vi "WriteHeader.vi"(0 "Path In":path, 1 "error in (no error)":errorcluster, 2 "Line 1":string, 3 "Line 2":string, 4 "Line 3":string, 5 "Line 4":string, 7 "Line 5":string, 8 "UTC format":bool, 9 "Line 6":string, 11 "Line 7":string, 13 "Line 8":string, 18 "Line 10":string, 19 "Line 9":string) -> (14 "Path":path, 17 "error out":errorcluster)   [LabVIEW 2009]
doc: "This VI takes a file path (required) and appends a 10 line header. Each line of the header can be specified separately.\nLines are first run through the Format Date String VI, so entries such as %H:%M will be interpreted correctly. This VI is an important part of \"StartLogfile.vi\""
uses:
  <vilib>/Utility/file.llb/Write To Spreadsheet File (string).vi
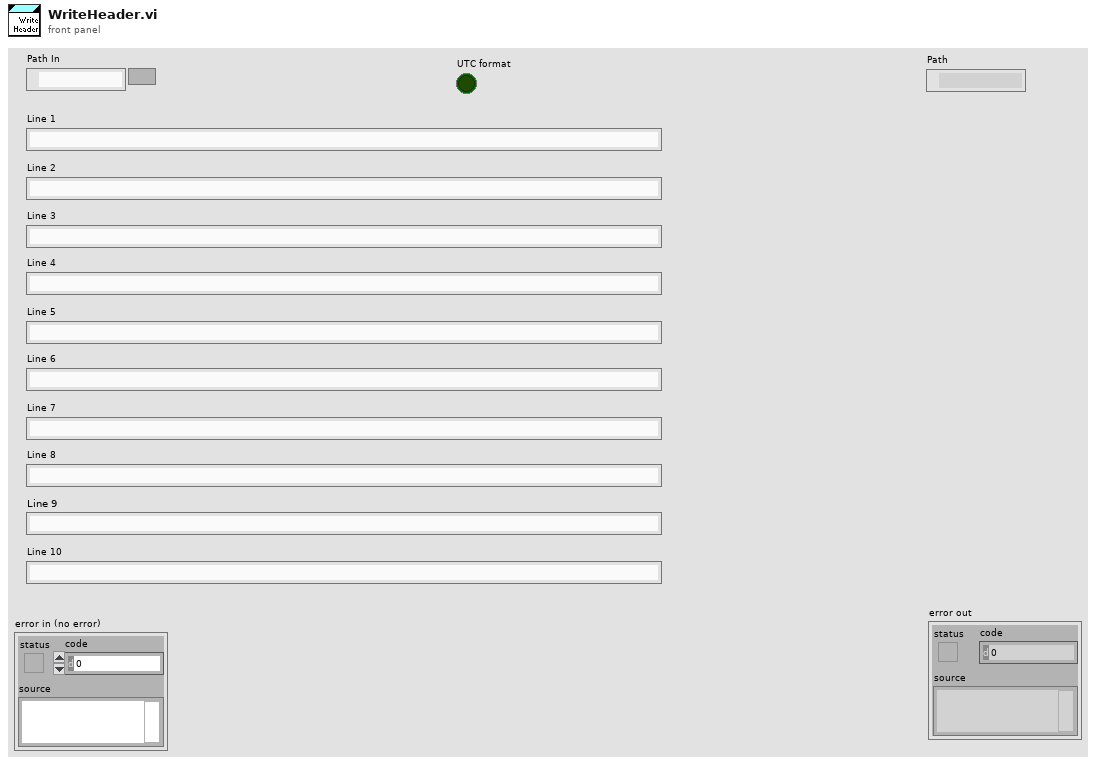
[diagram p1: front panel]
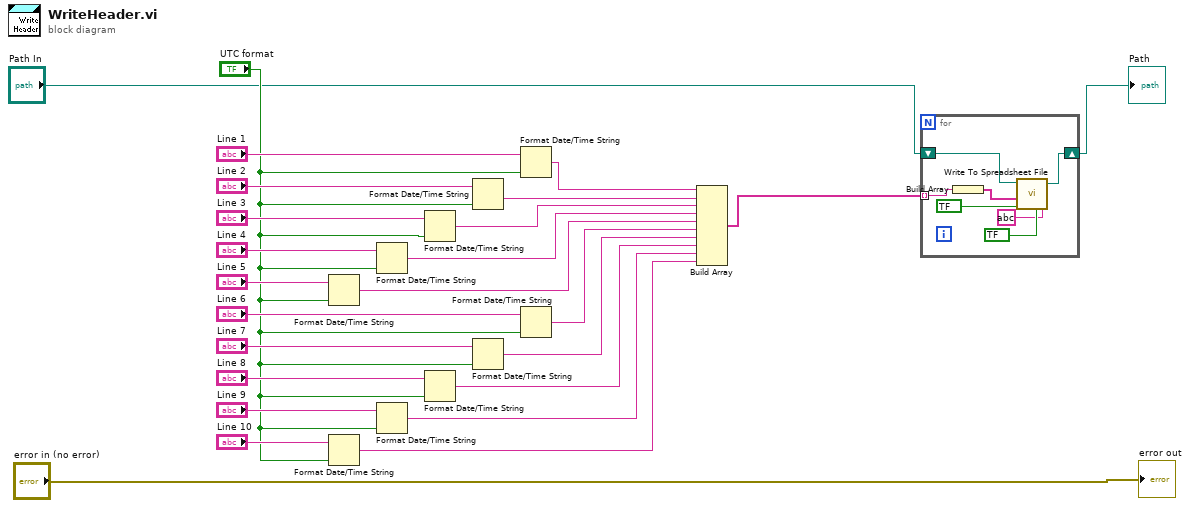
[diagram p0: block diagram]
diagram:
  n1 = Format Date/Time String(time format string (%c)="Line 5", UTC format="UTC format") -> (date/time string=w9:string)  [unwired: 1 in]
  n2 = Format Date/Time String(time format string (%c)="Line 10", UTC format="UTC format") -> (date/time string=w4:string)  [unwired: 1 in]
  n3 = Format Date/Time String(time format string (%c)="Line 4", UTC format="UTC format") -> (date/time string=w10:string)  [unwired: 1 in]
  n4 = Format Date/Time String(time format string (%c)="Line 9", UTC format="UTC format") -> (date/time string=w5:string)  [unwired: 1 in]
  n5 = Format Date/Time String(time format string (%c)="Line 3", UTC format="UTC format") -> (date/time string=w11:string)  [unwired: 1 in]
  n6 = Format Date/Time String(time format string (%c)="Line 8", UTC format="UTC format") -> (date/time string=w6:string)  [unwired: 1 in]
  n7 = Format Date/Time String(time format string (%c)="Line 2", UTC format="UTC format") -> (date/time string=w12:string)  [unwired: 1 in]
  n8 = Format Date/Time String(time format string (%c)="Line 7", UTC format="UTC format") -> (date/time string=w7:string)  [unwired: 1 in]
  n9 = Format Date/Time String(time format string (%c)="Line 1", UTC format="UTC format") -> (date/time string=w13:string)  [unwired: 1 in]
  n10 = Format Date/Time String(time format string (%c)="Line 6", UTC format="UTC format") -> (date/time string=w8:string)  [unwired: 1 in]
  n11 = Build Array(w13, w12, w11, w10, w9, w8, w7, w6, w5, w4) -> (w3:string[])
  n12 = for {
    shift-right: [w31] -> w25
    shift-left: "Path In" -> [w30]
    tunnel: w3 -> [w28] mode=indexing
    n13 = Build Array(w28) -> (w27:string[])
    n14 = call-poly <vilib>:"Write To Spreadsheet File.vi"("delimiter (\\t)"=string ? ("delimiter (\\t)"), "transpose? (no:F)"=bool ?, "append to file? (new file:F)"=bool ?, "1D data"=w27, "file path (dialog if empty)"=w30) -> ("new file path (Not A Path if cancelled)"=w31:path)  [unwired: 3 in]
  }
  "Path" <- w25
  "error out" <- "error in (no error)"
